vi "Initialize From File.vi"(0 "CommitNIPKG_LV in":refnum<class "CommitNIPKG_LV.lvclass">, 11 "error in (no error)":errorcluster) -> (4 "CommitNIPKG_LV out":refnum<class "CommitNIPKG_LV.lvclass">, 15 "error out":errorcluster)   [LabVIEW 2017, in "CL_G3_VIComponentBuilder.lvlib" / "CommitNIPKG_LV.lvclass"]
doc: "Initializes the class from the configuration file."
uses:
  CommitNIPKG_LV.lvclass
  C:/builds/Component BuilderBT/SrcDist/Commit Behavior/Commit/Commit.lvclass
  Commit/Commit.lvclass/Commit.ctl
  CommitNIPKG_LV.lvclass/CommitNIPKG_LV.ctl
  Accessors/Write Commit Feed Folderpaths.vi
  Commit/Accessors/Read Commit Config File.vi
  Commit/Accessors/Read Exports Commit Destination Folder.vi
  Commit/Commit.lvclass
  <vilib>/Utility/config.llb/NI_LVConfig.lvlib
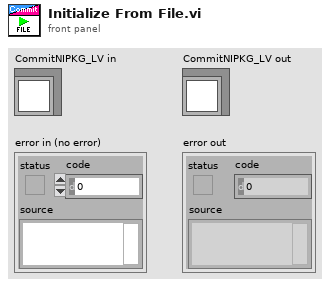
[diagram p1: front panel]
types:
  T1 = typedef "NI_LVConfig.lvlib/Config Data RefNum.ctl" = refnum<k1>
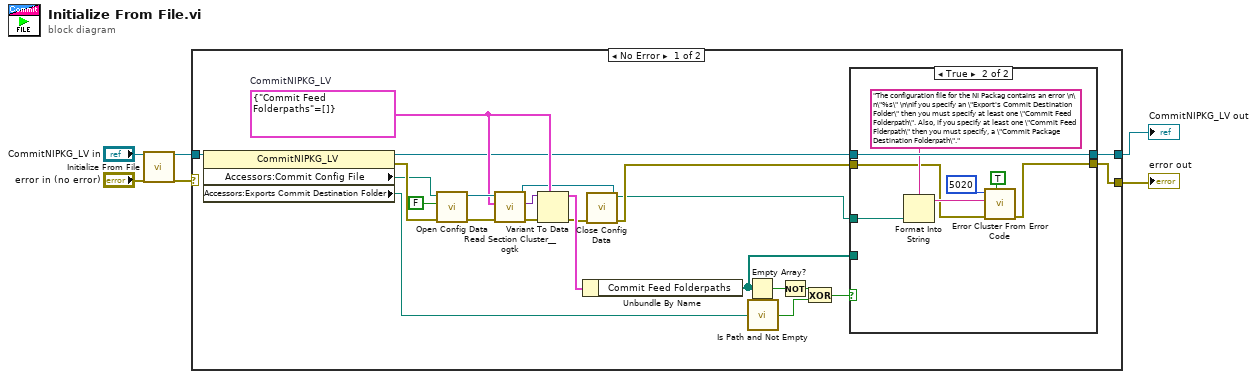
[diagram p0: block diagram]
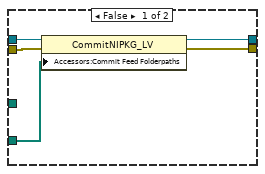
[diagram p2: hidden frame]
diagram:
  n1 = call-parent "Initialize From File.vi"("Commit in"="CommitNIPKG_LV in", "error in (no error)"="error in (no error)") -> ("Commit out"=w4:refnum<class "CommitNIPKG_LV.lvclass">, "error out"=w3:errorcluster)  [unwired: 12 in]
  n2 = case shown="No Error" w3 {
    selector: w3 -> [_ w44]
    tunnel: [w28 w44] -> w1
    tunnel: [w29 w43] -> w2
    tunnel: w4 -> [w27 w43]
    frame No Error {
      w23 = cluster{"Commit Feed Folderpaths":path[]} {"Commit Feed Folderpaths"=[]}  # CommitNIPKG_LV
      n3 = property class="CommitNIPKG_LV"(reference=w27) -> (reference out=w10:refnum<class "CommitNIPKG_LV.lvclass">, error out=w19:errorcluster, "Accessors:Commit Config File"=w18:path, "Accessors:Exports Commit Destination Folder"=w7:path)  [unwired: 1 in]
      n4 = call <vilib>:"Open Config Data.vi"("error in (no error)"=w19, "create file if necessary (T)"=FALSE, "configuration file path"=w18) -> ("error out"=w21:errorcluster, "refnum"=w25:T1)  [unwired: 6 in, 1 out]
      n5 = call <userlib>:"Read Section Cluster__ogtk.vi"("error in (no error)"=w21, "Section Formatted Cluster Type"=w23, "refnum"=w25) -> ("error out"=w20:errorcluster, "Section Formatted Cluster"=w24:variant, "dup refnum"=w17:T1)  [unwired: 4 in, 2 out]
      n6 = Variant To Data(error in=w20, type=w23, Variant=w24) -> (data=w22:cluster{"Commit Feed Folderpaths":path[]}, error out=w16:errorcluster)
      n7 = Unbundle By Name(w22) -> ("Commit Feed Folderpaths"=w15:path[])
      n8 = call <vilib>:"Close Config Data.vi"("error in (no error)"=w16, "refnum"=w17) -> ("error out"=w9:errorcluster, "file path"=w8:path)  [unwired: 8 in]
      n9 = Empty Array?(array=w15) -> (empty?=w14:bool)
      n10 = call <vilib>:"Is Path and Not Empty.vi"("path"=w7) -> ("Is Path and Not Empty?"=w13:bool)  [unwired: 4 in]
      n11 = Not(x=w14) -> (.not. x?=w11:bool)
      n12 = Exclusive Or(1:w13, 2:w11) -> (0:w12:bool)
      n13 = case shown="True" w12 {
        tunnel: [w34 w42] -> w29
        tunnel: [w33 w37] -> w28
        tunnel: w10 -> [w32 w42]
        tunnel: w15 -> [w31 _]
        tunnel: w8 -> [_ w40]
        tunnel: w9 -> [w30 w35]
        frame False {
          n14 = property class="CommitNIPKG_LV"(reference=w32, error in=w30, "Accessors:Commit Feed Folderpaths"=w31) -> (reference out=w34:refnum<class "CommitNIPKG_LV.lvclass">, error out=w33:errorcluster)
        }
        frame True {
          n15 = Format Into String(format string="The configuration file for the NI Packag contains an error \n\n\"%s\" \n\nIf you specify an \"Export's Commit Destination Folder\" then you must specify at least one \"Commit Feed Folderpath\". Also, if you specify at least one \"Commit Feed Flderpath\" then you must specify, a \"Commit Package Destination Folderpath\".", w40) -> (resulting string=w38:string)  [unwired: 2 in, 1 out]
          n16 = call <vilib>:"Error Cluster From Error Code.vi"("show call chain? (False)"=TRUE, "error in (no error)"=w35, "error message (\"\")"=w38, "error code (0)"=5020) -> ("error out"=w37:errorcluster)  [unwired: 5 in]
        }
      }
    }
    frame Error {
    }
  }
  "error out" <- w1
  "CommitNIPKG_LV out" <- w2
